vi "Invert.vi"(10 "Invert Colors":bool, 11 "Refnum in":T1) -> (3 "Refnum out":T1)   [LabVIEW 2018]
uses:
  <vilib>/vision/Image Controls.llb/IMAQ Image.ctl
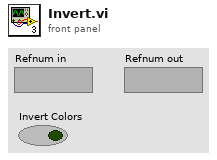
[diagram p1: front panel]
types:
  T1 = typedef "IMAQ Image.ctl" = refnum<image>
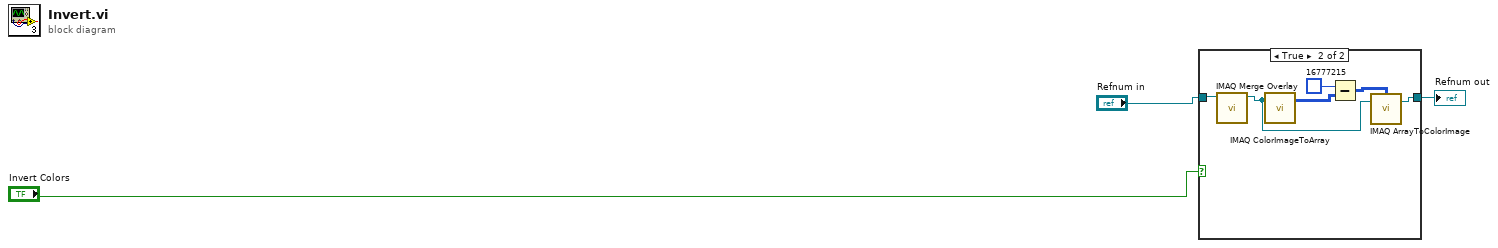
[diagram p0: block diagram]
diagram:
  n1 = case shown="True" "Invert Colors" {
    tunnel: [w4 w9] -> w2
    tunnel: "Refnum in" -> [w4 w5]
    frame False {
    }
    frame True {
      n2 = call "IMAQ Merge Overlay"("Image Src"=w5) -> ("Image Dst Out"=w6:T1)  [unwired: 9 in, 1 out]
      n3 = call "IMAQ ColorImageToArray"("Image"=w6) -> ("Image Pixels (U32)"=w10:u32[][])  [unwired: 3 in, 2 out]
      n4 = Subtract(x=u32 16777215, y=w10) -> (x-y=w8:u32[][])
      n5 = call "IMAQ ArrayToColorImage"("Image Pixels (U32)"=w8, "Image"=w6) -> ("Image Out"=w9:T1)  [unwired: 3 in, 1 out]
    }
  }
  "Refnum out" <- w2
